vi "1L13-tb-conv-tb2D-en-tb1D.vi"(1 "tb 2D":dbl[][](array[numeric])) -> (0 "tb 1D":dbl[](array[numeric]))   [LabVIEW 2010, in "lv_01.lvlib"]
uses:
  lv_01.lvlib
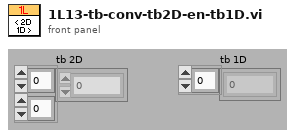
[diagram p1: front panel]
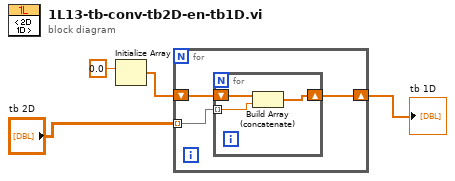
[diagram p0: block diagram]
diagram:
  n1 = Initialize Array(0.0 ("élément")) -> (w3:dbl[])  [unwired: 1 in]
  n2 = for {
    tunnel: "tb 2D" -> [w7] mode=indexing
    shift-right: [w5] -> w4
    shift-left: w3 -> [w6]
    n3 = for {
      tunnel: w7 -> [w10] mode=indexing
      shift-right: [w8] -> w5
      shift-left: w6 -> [w9]
      n4 = Build Array (concatenate)(w9, w10) -> (w8:dbl[])
    }
  }
  "tb 1D" <- w4
